vi "Open Connection--SubVI.vi"(8 "error in (no error)":errorcluster, 10 "VISA Refnum in":refnum<visa-resource-name>, 11 "Watlow F4T in":refnum<class "Watlow F4T.lvclass">) -> (0 "error out":errorcluster, 2 "IsConnected":bool, 3 "Watlow F4T out":refnum<class "Watlow F4T.lvclass">)   [LabVIEW 2024, in "Watlow F4T.lvclass"]
uses:
  Watlow F4T.lvclass
  Watlow F4T.lvclass/Watlow F4T.ctl
  <instrlib>/Watlow Std Bus/Public/Watbus.dll
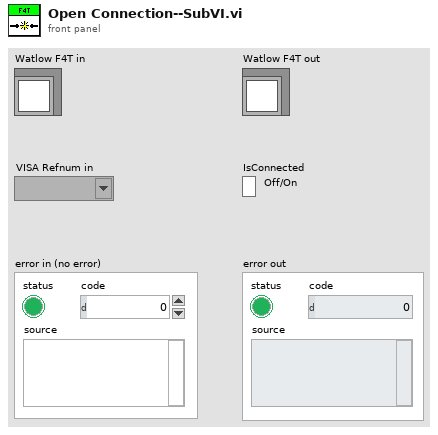
[diagram p1: front panel]
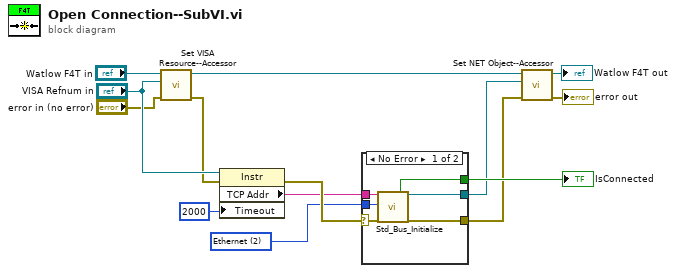
[diagram p0: block diagram]
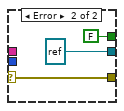
[diagram p2: hidden frame]
diagram:
  w11 = 2 items=["Usb", "Serial", "Ethernet", "Unconnected"] ("InterfaceType")
  n1 = call-dynamic "Set VISA Resource--Accessor.vi"("error in (no error)"="error in (no error)", "VISA Resource"="VISA Refnum in", "Watlow F4T in"="Watlow F4T in") -> ("error out"=w6:errorcluster, "Watlow F4T out"=w4:refnum<class "Watlow F4T.lvclass">)  [unwired: 7 in]
  n2 = property class="Instr"(reference="VISA Refnum in", error in=w6, "Timeout"=u32 2000 ("General Settings:Timeout Value")) -> (error out=w14:errorcluster, "TCP Addr"=w10:string)  [unwired: 1 out]
  n3 = case shown="No Error" w14 {
    selector: w14 -> [w15 w23]
    tunnel: w10 -> [w20 _]
    tunnel: w11 -> [w19 _]
    tunnel: [w18 FALSE ("IsConnected")] -> w12
    tunnel: [w17 w23] -> w5
    tunnel: [w16 refnum<k24> refnum ("ILabVIEW")] -> w3
    frame No Error {
      n4 = call <instrlib>:"Std_Bus_Initialize.vi"("Communications Port"=w20, "InterfaceType"=w19, "error in (no error)"=w15) -> ("IsConnected"=w18:bool, "ILabVIEW"=w16:refnum<k24>, "error out"=w17:errorcluster)  [unwired: 14 in]
    }
    frame Error {
    }
  }
  "IsConnected" <- w12
  n5 = call "Set NET Object--Accessor.vi"("error in (no error)"=w5, ".NET Object"=w3, "Watlow F4T in"=w4) -> ("error out"=→"error out":errorcluster, "Watlow F4T out"=→"Watlow F4T out":refnum<class "Watlow F4T.lvclass">)  [unwired: 7 in]
